vi "delta_3st.vi"(8 "d":dbl, 9 "c":dbl, 10 "b":dbl, 11 "a":dbl) -> (1 "q":dbl, 2 "p":dbl, 3 "Delta trzeciego stopnia":dbl)   [LabVIEW 2020]
doc: "Obliczanie wyróżnika wielomianu ze wzoru"
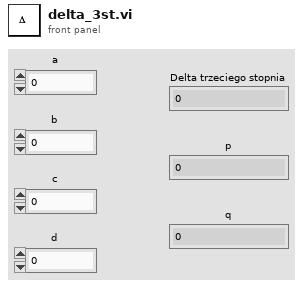
[diagram p1: front panel]
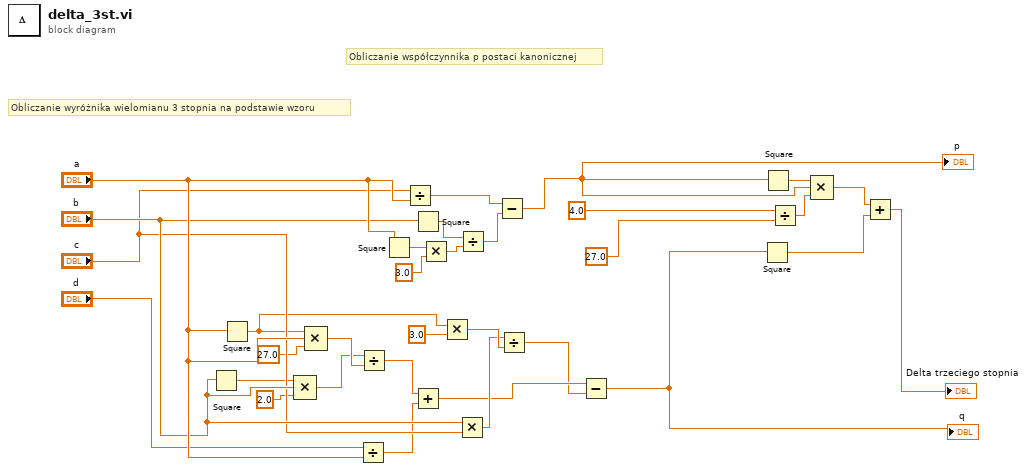
[diagram p0: block diagram]
diagram:
  # "Obliczanie współczynnika p postaci kanonicznej"
  # "Obliczanie wyróżnika wielomianu 3 stopnia na podstawie wzoru"
  n1 = Square(x="b") -> (x^2=w13:dbl)
  n2 = Square(x="a") -> (x^2=w5:dbl)
  n3 = Compound Arithmetic op=MULTIPLY(w13, "b", 2.0 ("value")) -> (w9:dbl)
  n4 = Compound Arithmetic op=MULTIPLY(w5, "a", 27.0 ("value")) -> (w10:dbl)
  n5 = Divide(x="d", y="a") -> (x/y=w7:dbl)
  n6 = Divide(x=w9, y=w10) -> (x/y=w8:dbl)
  n7 = Square(x="a") -> (x^2=w14:dbl)
  n8 = Divide(x="c", y="a") -> (x/y=w16:dbl)
  n9 = Square(x="b") -> (x^2=w15:dbl)
  n10 = Add(x=w8, y=w7) -> (x+y=w2:dbl)
  n11 = Multiply(x=w14, y=3.0) -> (x*y=w18:dbl)
  n12 = Multiply(x=w5, y=3.0 ("value")) -> (x*y=w4:dbl)
  n13 = Multiply(x="b", y="c") -> (x*y=w3:dbl)
  n14 = Divide(x=w15, y=w18) -> (x/y=w17:dbl)
  n15 = Subtract(x=w16, y=w17) -> (x-y=w26:dbl)
  "p" <- w26
  n16 = Divide(x=w3, y=w4) -> (x/y=w1:dbl)
  n17 = Subtract(x=w2, y=w1) -> (x-y=w25:dbl)
  "q" <- w25
  n18 = Square(x=w25) -> (x^2=w32:dbl)
  n19 = Square(x=w26) -> (x^2=w27:dbl)
  n20 = Divide(x=4.0, y=27.0 ("x")) -> (x/y=w30:dbl)
  n21 = Compound Arithmetic op=MULTIPLY(w27, w26, w30) -> (w31:dbl)
  n22 = Add(x=w31, y=w32) -> (x+y=→"Delta trzeciego stopnia":dbl)
